vi "NewCore.vi"(8 "error in (no error)":errorcluster, 10 "ParamsArray":variant[](array[variant]), 11 "ConcreteCreatorA in":refnum<class "ConcreteCreatorA.lvclass">) -> (0 "error out":errorcluster, 3 "ConcreteCreatorA out":refnum<class "ConcreteCreatorA.lvclass">)   [LabVIEW 2020, in "FactoryMethod.lvlib" / "ConcreteCreatorA.lvclass"]
uses:
  ConcreteCreatorA.lvclass
  Private/TypeDef/privateData.ctl
  ConcreteCreatorA.lvclass/ConcreteCreatorA.ctl
  Creator/Creator.lvclass
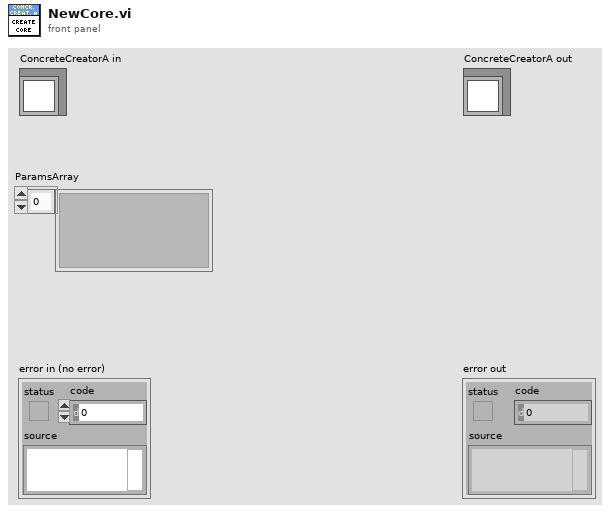
[diagram p1: front panel]
types:
  T1 = typedef "FactoryMethod.lvlib/ConcreteCreatorA.lvclass/privateData.ctl" = cluster{"Dummy":i32}
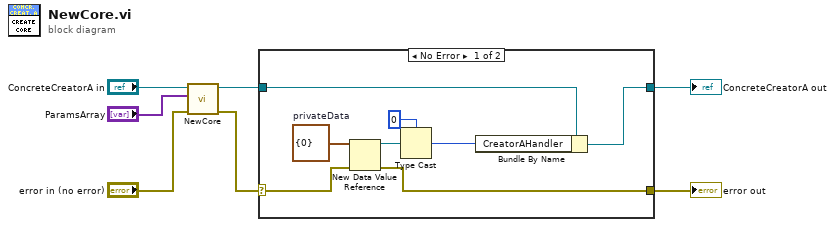
[diagram p0: block diagram]
diagram:
  n1 = call-parent "NewCore.vi"("error in (no error)"="error in (no error)", "ParamsArray"="ParamsArray", "Creator in"="ConcreteCreatorA in") -> ("error out"=w2:errorcluster, "Creator out"=w5:refnum<class "ConcreteCreatorA.lvclass">)  [unwired: 7 in]
  n2 = case shown="No Error" w2 {
    selector: w2 -> [w9 w17]
    tunnel: [w10 w17] -> w3
    tunnel: [w12 w16] -> w4
    tunnel: w5 -> [w11 w16]
    frame No Error {
      w8 = T1 {"Dummy"=0}  # privateData
      n3 = New Data Value Reference(data value=w8, error in=w9) -> (data value reference=w15:refnum<data-value>, error out=w10:errorcluster)
      n4 = Type Cast(type=u32 0, x=w15) -> (*(type *) &x=w13:u32)
      n5 = Bundle By Name(cluster=w11, "CreatorAHandler"=w13) -> (w12:refnum<class "ConcreteCreatorA.lvclass">)
    }
    frame Error {
    }
  }
  "error out" <- w3
  "ConcreteCreatorA out" <- w4
